vi "Test Pi Speed.vi"() -> ()   [LabVIEW 2020]
uses:
  Labview Library/Libraries/HW_PI/E-727/PI E-727 Module/Axis.ctl
  <vilib>/Analysis/baseanly.llb/Mean (DBL).vi
  Labview Library/Libraries/HW_PI/E-727/PI E-727 Module/PI E-727 Module.lvlib
  <vilib>/Analysis/NI_AALBase.lvlib
panel:
  out "Waveform Chart":dbl(graph)
  in  "stop":bool
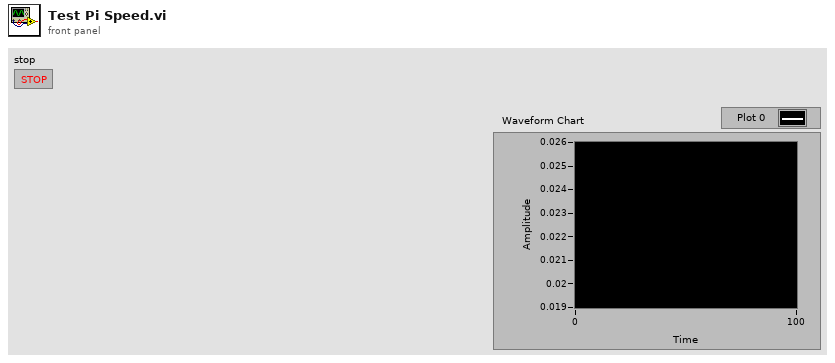
[diagram p1: front panel]
types:
  T1 = typedef "PI E-727 Module.lvlib/Axis.ctl" = enum16{"X", "Y", "Z"}
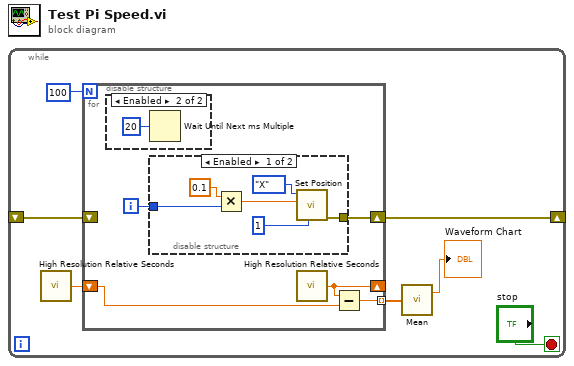
[diagram p0: block diagram]
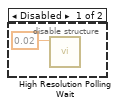
[diagram p2: hidden frame]
diagram:
  n1 = while {
    shift-right: [w6] -> _
    shift-left: _ -> [w5]
    stop <- "stop" stop-if-true
    n2 = call <vilib>:"High Resolution Relative Seconds.vi"() -> ("relative seconds"=w3:dbl)
    n3 = for {
      N: 100 -> [_]
      shift-right: [w11] -> w6
      shift-left: w5 -> [_]
      shift-right: [w10] -> _
      shift-left: w3 -> [w9]
      tunnel: [w8] -> w2 mode=indexing
      i -> [w12]
      n4 = disable-structure shown="Enabled" {
        frame Disabled {
          n5 = call <vilib>:"High Resolution Polling Wait.vi"("seconds to wait"=0.02) -> ()  [unwired: 10 in, 1 out]
        }
        frame Enabled {
          n6 = Wait Until Next ms Multiple(millisecond multiple=u32 20) -> ()  [unwired: 1 out]
        }
      }
      n7 = disable-structure shown="Enabled" {
        disable-tunnel: w12 -> [w20 _]
        disable-tunnel: [w16 _] -> w11
        frame Enabled {
          n8 = Multiply(x=0.1, y=w20) -> (x*y=w18:dbl)
          n9 = call "Set Position.vi"("Idle After Moving (ms)"=1, "Position"=w18, "Axis"=Axis."X") -> ("error out"=w16:errorcluster)  [unwired: 8 in]
        }
        frame Disabled {
        }
      }
      n10 = call <vilib>:"High Resolution Relative Seconds.vi"() -> ("relative seconds"=w10:dbl)
      n11 = Subtract(x=w10, y=w9) -> (x-y=w8:dbl)
    }
    n12 = call-poly <vilib>:"Mean.vi"("X"=w2) -> ("mean"=→"Waveform Chart":dbl)  [unwired: 1 out]
  }
